vi "GEOM_VAR_GeomModifiers.vi"(9 "Action":T4, 10 "GEOM_modifiers":T1={"Binning"={"x"=1, "y"=1}, "sections"=[]} {"Binning"."y" min=1; "Binning"."x" min=1}) -> (2 "GEOM_modifiers out":T1={"Binning"={"x"=1, "y"=1}, "sections"=[]} {"Binning"."y" min=1; "Binning"."x" min=1})   [LabVIEW 2016]
uses:
  GEOM_VAR_action.ctl
  GEOM_AmpModifiers.ctl
  GEOM_Binning.ctl
  GEOM_Moifier.ctl
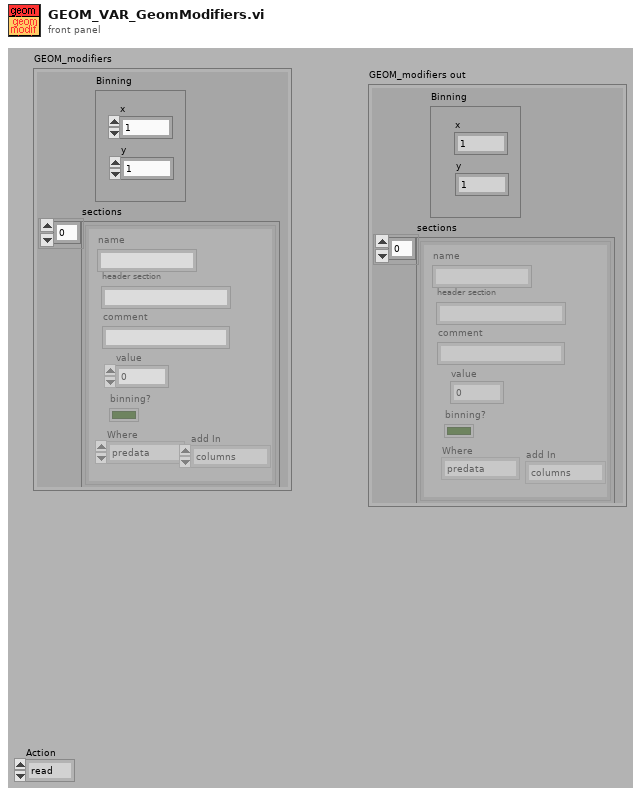
[diagram p1: front panel]
types:
  T1 = typedef "GEOM_AmpModifiers.ctl" = cluster{"Binning":T2, "sections":T3[]}
  T2 = typedef "GEOM_Binning.ctl" = cluster{"x":u32, "y":u32}
  T3 = typedef "GEOM_Moifier.ctl" = cluster{"name":string, "header section":string, "comment":string, "value":i32, "binning?":bool, "Where":enum16{"predata", "postdata"}, "add In":enum16{"columns", "rows", "none"}}
  T4 = typedef "GEOM_VAR_action.ctl" = enum16{"read", "write"}
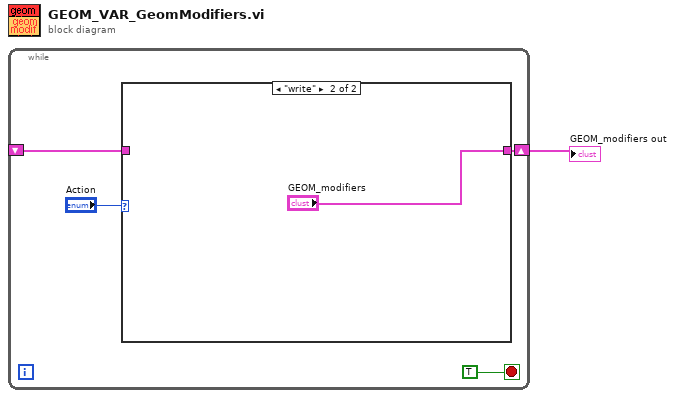
[diagram p0: block diagram]
diagram:
  n1 = while {
    shift-right: [w4] -> w1
    shift-left: _ -> [w3]
    stop <- TRUE stop-if-true
    n2 = case shown="\"write\"" "Action" {
      tunnel: [w6 "GEOM_modifiers"] -> w4
      tunnel: w3 -> [w6 _]
      frame "read", Default {
      }
      frame "write" {
      }
    }
  }
  "GEOM_modifiers out" <- w1
